vi "ziGetValueDemodSample.vi"(4 "error in":errorcluster, 5 "Demod Sample In":T1={"Timestamps (ticks)"=0, "X (Vrms)"=nan, "Y (Vrms)"=nan, "Osc Phase (deg)"=nan, "Freq (Hz)"=nan, "DIO"=0, "AuxIn0 (V)"=nan, "AuxIn1 (V)"=nan, "Trigger"=0}, 6 "Path":string, 7 "Handle In":T2 {"Handle" format="0x%08x"; "Conn" format="0x%08x"}) -> (0 "error out":errorcluster, 1 "Demod Sample Out":T1, 3 "Handle Out":T2 {"Handle" format="0x%08x"; "Conn" format="0x%08x"})   [LabVIEW 2009, in "Zurich Instruments LabOne.lvlib"]
doc: "This function retrieves the newest available sample from a demodulator's sample node. The value first found is returned if more than one value is available (a wildcard is used in the path). This function is only applicable to paths matching DEMODS/[0-9]+/SAMPLE."
uses:
  <instrlib>/Zurich Instruments LabOne/Zurich Instruments LabOne.lvlib
  <instrlib>/Zurich Instruments LabOne/Public/ziTypeHandle.ctl
  <instrlib>/Zurich Instruments LabOne/Public/Data/ziTypeDemodSampleSingle.ctl
  <instrlib>/Zurich Instruments LabOne/Private/ziLV32.dll
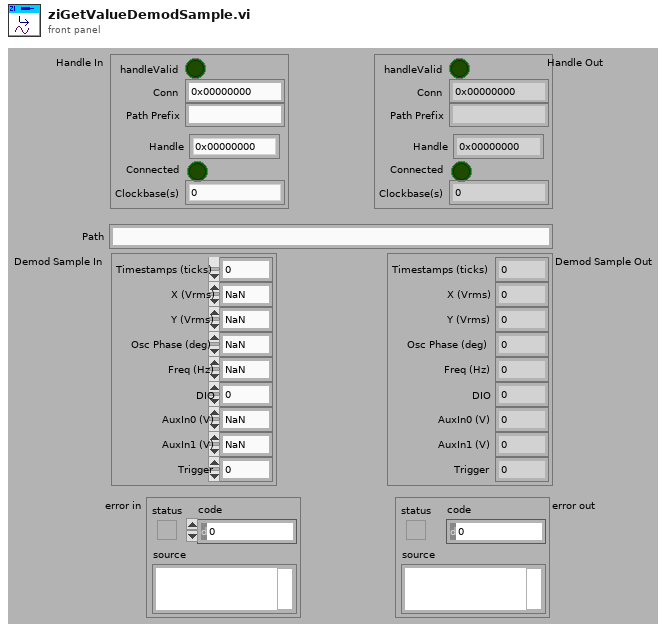
[diagram p1: front panel]
types:
  T1 = typedef "Zurich Instruments LabOne.lvlib/ziTypeDemodSampleSingle.ctl" = cluster{"Timestamps (ticks)":u64, "X (Vrms)":dbl, "Y (Vrms)":dbl, "Osc Phase (deg)":dbl, "Freq (Hz)":dbl, "DIO":u32, "AuxIn0 (V)":dbl, "AuxIn1 (V)":dbl, "Trigger":u32}
  T2 = typedef "Zurich Instruments LabOne.lvlib/ziTypeHandle.ctl" = cluster{"handleValid":bool, "Conn":u64, "Path Prefix":string, "Handle":u64, "Connected":bool, "Clockbase(s)":dbl}
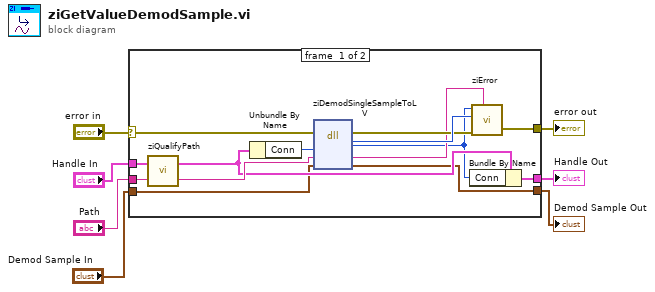
[diagram p0: block diagram]
diagram:
  n1 = case shown="No Error" "error in" {
    selector: "error in" -> [w12 w23]
    tunnel: [w10 w23] -> w6
    tunnel: [w18 w24] -> w5
    tunnel: "Handle In" -> [w16 w24]
    tunnel: [w9 w22] -> w7
    tunnel: "Demod Sample In" -> [w11 w22]
    tunnel: "Path" -> [w8 _]
    frame #0 {
      n2 = call <instrlib>:"ziQualifyPath.vi"("Path In"=w8, "Handle In"=w16) -> ("Path Out"=w17:string, "Handle Out"=w15:T2)
      n3 = Unbundle By Name(w15) -> ("Conn"=w21:u64)
      n4 = dll-call lib="C:/Program Files (x86)/National Instruments/LabVIEW 2009/instr.lib/Zurich Instruments LabOne/Private/ziLV*.*" fn="ziDemodSingleSampleToLV" label="ziAPIGetDemodSample"(error in=w12, "Conn"=w21, "Path"=w17, w11) -> (error out=w19:errorcluster, "return type"=w20:u32, "Conn"=w13:u64, "Path"=w14:string, w9:T1)  [unwired: 2 in, 1 out]
      n5 = Bundle By Name(cluster=w15, "Conn"=w13) -> (w18:T2)
      n6 = call <instrlib>:"ziError.vi"("Conn"=w13, "ziErrorCode"=w20, "Error In"=w19, "Annotation"=w14) -> ("Error Out"=w10:errorcluster)  [unwired: 1 in, 1 out]
    }
    frame #1 {
    }
  }
  "Handle Out" <- w5
  "error out" <- w6
  "Demod Sample Out" <- w7
